vi "Preview Waveforms.vi"(8 "Change in Time":dbl, 9 "In Use Cluster":T2, 10 "Input Read Data":dbl[][](array[numeric]), 11 "Input Decimated Data":dbl[][](array[numeric])) -> (1 "Output Waveform Cluster":T1, 3 "Output Data":dbl[][](array[numeric]))   [LabVIEW 2014]
panel:
  # "Preview Waveforms VI"
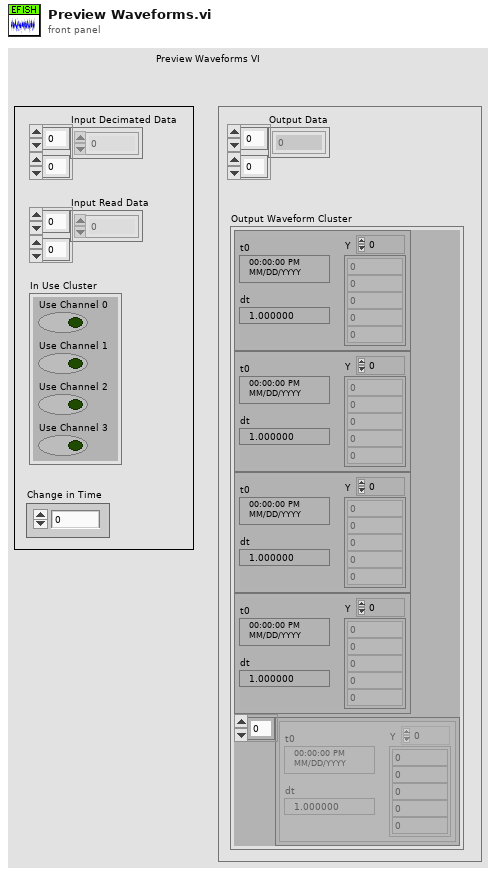
[diagram p1: front panel]
types:
  T1 = cluster{"Waveform":waveform(dbl), "Waveform":waveform(dbl), "Waveform":waveform(dbl), "Waveform":waveform(dbl), waveform(dbl)[]}
  T2 = cluster{"Use Channel 0":bool, "Use Channel 1":bool, "Use Channel 2":bool, "Use Channel 3":bool}
  T3 = cluster{waveform(dbl), waveform(dbl), waveform(dbl), waveform(dbl), waveform(dbl)[]}
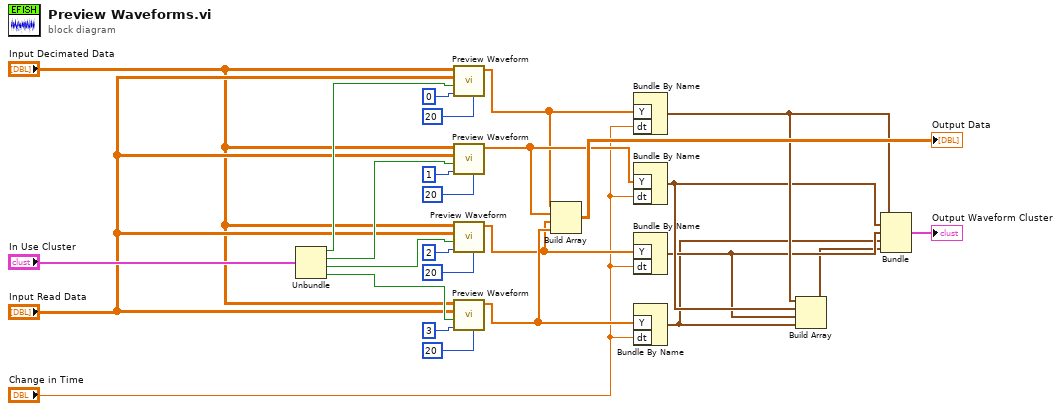
[diagram p0: block diagram]
diagram:
  n1 = Unbundle("In Use Cluster") -> ("Use Channel 0"=w19:bool, "Use Channel 1"=w20:bool, "Use Channel 2"=w21:bool, "Use Channel 3"=w22:bool)
  n2 = call "Preview Waveform.vi"("Decimation Multiple"=u16 20, "Channel #"=i8 0, "In Use?"=w19, "New Y Values"="Input Read Data", "Old Y Values"="Input Decimated Data") -> ("Output Y Values"=w23:dbl[])  [unwired: 6 in]
  n3 = call "Preview Waveform.vi"("Decimation Multiple"=u16 20, "Channel #"=i8 1, "In Use?"=w20, "New Y Values"="Input Read Data", "Old Y Values"="Input Decimated Data") -> ("Output Y Values"=w24:dbl[])  [unwired: 6 in]
  n4 = call "Preview Waveform.vi"("Decimation Multiple"=u16 20, "Channel #"=i8 2, "In Use?"=w21, "New Y Values"="Input Read Data", "Old Y Values"="Input Decimated Data") -> ("Output Y Values"=w25:dbl[])  [unwired: 6 in]
  n5 = call "Preview Waveform.vi"("Decimation Multiple"=u16 20, "Channel #"=i8 3, "In Use?"=w22, "New Y Values"="Input Read Data", "Old Y Values"="Input Decimated Data") -> ("Output Y Values"=w26:dbl[])  [unwired: 6 in]
  n6 = Build Array(w23, w24, w25, w26) -> (→"Output Data":dbl[][])
  n7 = Bundle By Name("Y"=w23, "dt"="Change in Time") -> (w7:waveform(dbl))  [unwired: 1 in]
  n8 = Bundle By Name("Y"=w24, "dt"="Change in Time") -> (w6:waveform(dbl))  [unwired: 1 in]
  n9 = Bundle By Name("Y"=w25, "dt"="Change in Time") -> (w5:waveform(dbl))  [unwired: 1 in]
  n10 = Bundle By Name("Y"=w26, "dt"="Change in Time") -> (w4:waveform(dbl))  [unwired: 1 in]
  n11 = Build Array(w7, w6, w5, w4) -> (w3:waveform(dbl)[])
  n12 = Bundle(w7, w6, w5, w4, w3) -> (→"Output Waveform Cluster":T3)  [unwired: 1 in]
